vi "Python@SetCaptureFile__Parameter.vi"(1 "ParamterIn":string) -> (0 "ParamterOut":string)   [LabVIEW 2020]
uses:
  MainFrame/Global.vi
panel:
  out "Image":T1(plugin-control)
  in  "Picture":string(combo)
  in  "PythonName":string(combo)="750"
  in  "CamName":string(combo)
  in  "Confirm":bool
  # "Python@SetCaptureFile $Capture,$Picture,$PythonName"
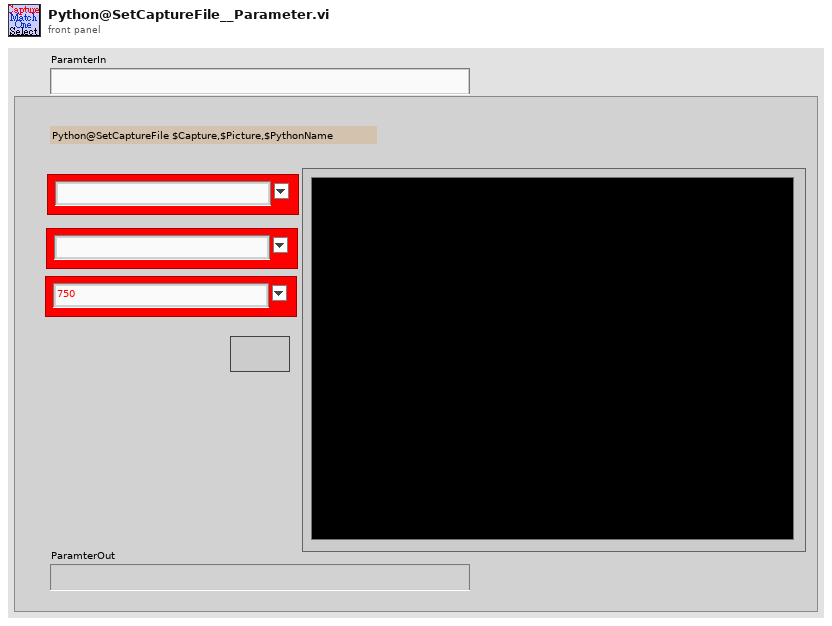
[diagram p1: front panel]
types:
  T1 = typedef "IMAQ Image.ctl" = refnum<image>
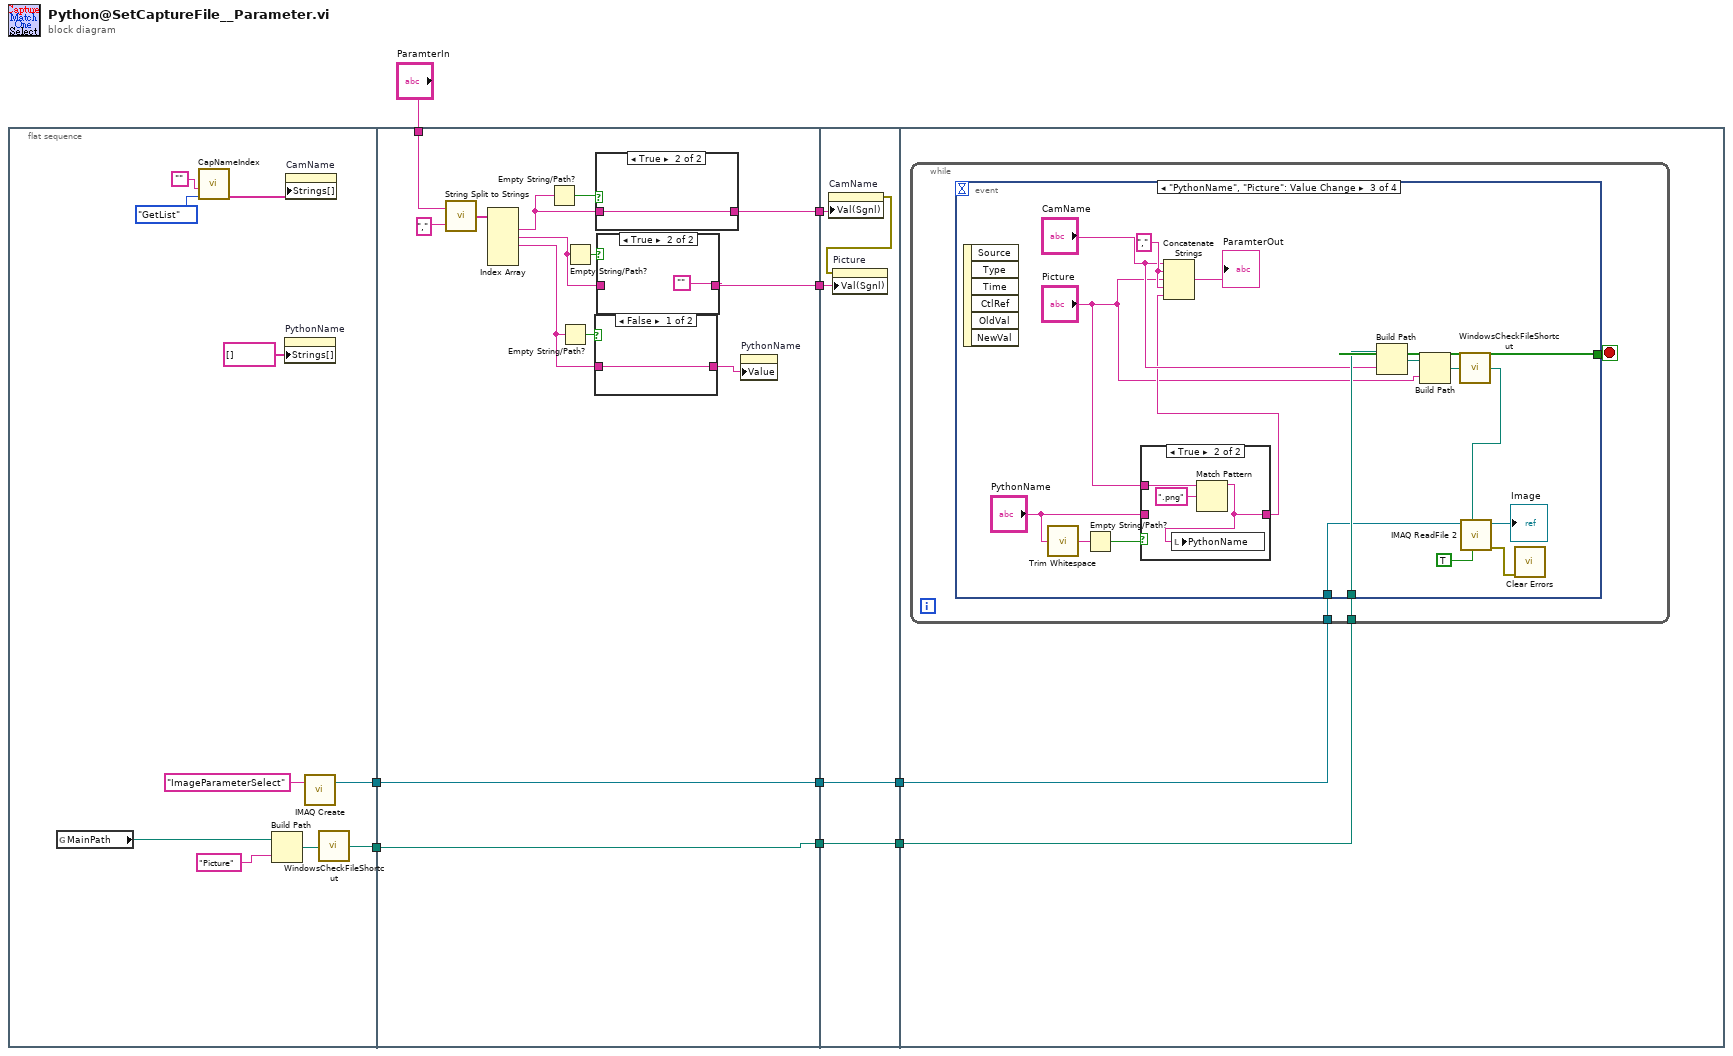
[diagram p0: block diagram]
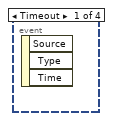
[diagram p5: hidden frame]
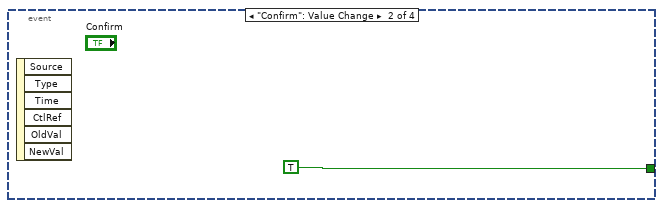
[diagram p6: hidden frame]
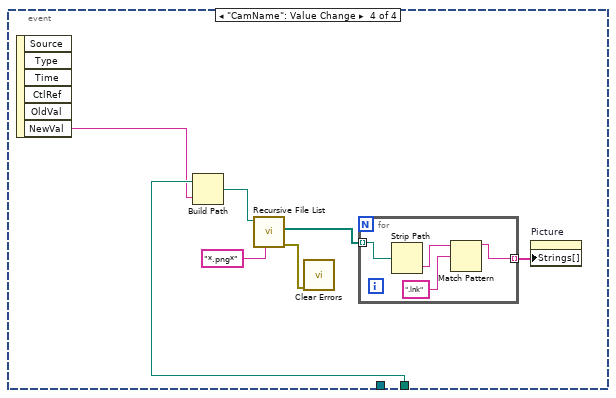
[diagram p8: hidden frame]
diagram:
  n1 = flat-sequence {
    tunnel: [w15] -> w8
    tunnel: [w10] -> w3
    tunnel: "ParamterIn" -> [w31]
    tunnel: w8 -> [w24]
    tunnel: [w24] -> w7
    tunnel: [w22] -> w4
    tunnel: w3 -> [w22]
    tunnel: [w21] -> w2
    tunnel: [w20] -> w1
    tunnel: w7 -> [w44]
    tunnel: [w44] -> w6
    tunnel: [w43] -> w5
    tunnel: w4 -> [w43]
    tunnel: w2 -> [w42]
    tunnel: w1 -> [w40]
    tunnel: w6 -> [w46]
    tunnel: w5 -> [w45]
    frame #0 {
      n2 = global read "Global.vi" "MainPath"() -> (w13:path)
      n3 = call "CapNameIndex.vi"("OP"=enum16{"AddCam", "GetIndex", "Init", "GetList"}."GetList", "CamName"="") -> ("DeviceList"=w18:string[])  [unwired: 2 in, 3 out]
      n4 = Build Path(base path=w13, name or relative path="Picture") -> (appended path=w11:path)
      n5 = property on="PythonName" class="CmbBox"("Strings[]"=string[] [] ("Strings []")) -> ()  [unwired: 2 in, 2 out]
      n6 = property on="CamName" class="CmbBox"("Strings[]"=w18) -> ()  [unwired: 2 in, 2 out]
      n7 = call "IMAQ Create"("Image Name"="ImageParameterSelect") -> ("New Image"=w15:T1)  [unwired: 4 in, 1 out]
      n8 = call "WindowsCheckFileShortcut.vi"("LinkPath"=w11) -> ("TargetPath"=w10:path)  [unwired: 4 in]
    }
    frame #1 {
      n9 = call "String Split to Strings.vi"("search string/char (-)"=",", "String"=w31) -> ("Array"=w33:string[])
      n10 = Index Array(array=w33) -> (element #1=w23:string, element #2=w25:string, element #3=w28:string)  [unwired: 5 in, 2 out]
      n11 = Empty String/Path?(string/path=w23) -> (empty?=w30:bool)
      n12 = Empty String/Path?(string/path=w28) -> (empty?=w29:bool)
      n13 = Empty String/Path?(string/path=w25) -> (empty?=w26:bool)
      n14 = case shown="False" w29 {
        tunnel: [w36 w37] -> w27
        tunnel: w28 -> [w36 w37]
        frame False {
        }
        frame True {
        }
      }
      n15 = case shown="True" w30 {
        tunnel: w23 -> [w38 w39]
        tunnel: [w38 w39] -> w20
        frame False {
        }
        frame True {
        }
      }
      n16 = case shown="True" w26 {
        tunnel: [w34 ""] -> w21
        tunnel: w25 -> [w34 _]
        frame False {
        }
        frame True {
        }
      }
      n17 = property on="PythonName" class="CmbBox"("Value"=w27) -> ()  [unwired: 2 in, 2 out]
    }
    frame #2 {
      n18 = property on="CamName" class="CmbBox"("Val(Sgnl)"=w40) -> (error out=w41:errorcluster)  [unwired: 2 in, 1 out]
      n19 = property on="Picture" class="CmbBox"(error in=w41, "Val(Sgnl)"=w42) -> ()  [unwired: 1 in, 2 out]
    }
    frame #3 {
      n20 = while {
        tunnel: w46 -> [w48]
        tunnel: w45 -> [w47]
        stop <- w49 stop-if-true
        n21 = event shown="[2] \"PythonName\", \"Picture\": Value Change" {
          selector: _ -> [_ _ _ _]
          dyn-events: _ -> [_ _ _ _]
          timeout: _ -> [_ _ _ _]
          tunnel: [_ TRUE _ _] -> w49
          tunnel: w48 -> [_ _ w54 _]
          tunnel: w47 -> [_ _ w64 w74]
          event Timeout {
            n22 = event-data() -> ()  [unwired: 1 in, 3 out]
          }
          event "Confirm": Value Change {
            n23 = event-data() -> ()  [unwired: 1 in, 6 out]
          }
          event "PythonName", "Picture": Value Change {
            w65 = "," ("string")
            n24 = event-data() -> ()  [unwired: 1 in, 6 out]
            n25 = call <vilib>:"Trim Whitespace.vi"("string"="PythonName") -> ("trimmed string"=w59:string)  [unwired: 1 in]
            n26 = Empty String/Path?(string/path=w59) -> (empty?=w58:bool)
            n27 = case shown="True" w58 {
              tunnel: "PythonName" -> [w67 _]
              tunnel: [w67 w68] -> w56
              tunnel: "Picture" -> [_ w70]
              frame False {
              }
              frame True {
                n28 = Match Pattern(string=w70, regular expression=".png") -> (before substring=w68:string)  [unwired: 1 in, 3 out]
                n29 = local write "PythonName"(w68) -> ()
              }
            }
            n30 = Concatenate Strings("CamName", w65, "Picture", w65, w56) -> (→"ParamterOut":string)
            n31 = Build Path(base path=w64, name or relative path="CamName") -> (appended path=w62:path)
            n32 = Build Path(base path=w62, name or relative path="Picture") -> (appended path=w52:path)
            n33 = call "WindowsCheckFileShortcut.vi"("LinkPath"=w52) -> ("TargetPath"=w51:path)  [unwired: 4 in]
            n34 = call "IMAQ ReadFile 2"("Use File Path Image Type"=TRUE, "File Path"=w51, "Image"=w54) -> ("error out"=w61:errorcluster, "Image Out"=→"Image":T1)  [unwired: 4 in, 3 out]
            n35 = call <vilib>:"Clear Errors.vi"("error in (no error)"=w61) -> ()  [unwired: 5 in, 2 out]
          }
          event "CamName": Value Change {
            n36 = event-data() -> ("NewVal"=w73:string)  [unwired: 1 in, 5 out]
            n37 = Build Path(base path=w74, name or relative path=w73) -> (appended path=w72:path)
            n38 = call <vilib>:"Recursive File List.vi"("pattern"="*.png*", "Folder Path"=w72) -> ("error out"=w71:errorcluster, "All Files in Dir"=w76:path[])  [unwired: 5 in, 3 out]
            n39 = call <vilib>:"Clear Errors.vi"("error in (no error)"=w71) -> ()  [unwired: 5 in, 2 out]
            n40 = for {
              tunnel: w76 -> [w81] mode=indexing
              tunnel: [w78] -> w77 mode=indexing
              n41 = Strip Path(path=w81) -> (name=w80:string)  [unwired: 1 out]
              n42 = Match Pattern(string=w80, regular expression=".lnk") -> (before substring=w78:string)  [unwired: 1 in, 3 out]
            }
            n43 = property on="Picture" class="CmbBox"("Strings[]"=w77) -> ()  [unwired: 2 in, 2 out]
          }
        }
      }
    }
  }
